vi "Corrected Flow Setpoint SI.vi"(7 "Set? (F:Read)":bool, 8 "Error In":errorcluster, 9 "Flow Setpoint (0 l/min)":dbl[unit], 10 "Channel (0)":i32, 11 "VISA resource name":refnum<visa-resource-name>) -> (0 "Error Out":errorcluster, 1 "Flow Setpoint out":dbl[unit], 3 "dup VISA resource name":refnum<visa-resource-name>)   [LabVIEW 2011, in "MGC647C.lvlib"]
doc: "Read/Set corrected flow setpoint of a channel in SI unit."
uses:
  <instrlib>/MGC647C/MGC647C.lvlib
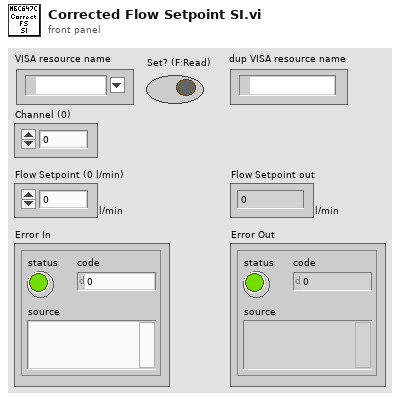
[diagram p1: front panel]
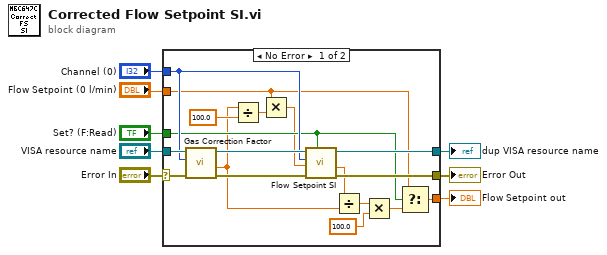
[diagram p0: block diagram]
diagram:
  n1 = case shown="No Error" "Error In" {
    selector: "Error In" -> [w25 w28]
    tunnel: "VISA resource name" -> [w26 w27]
    tunnel: [w21 w27] -> w7
    tunnel: [w20 w28] -> w6
    tunnel: "Set? (F:Read)" -> [w19 _]
    tunnel: "Flow Setpoint (0 l/min)" -> [w15 w29]
    tunnel: [w18 w29] -> w2
    tunnel: "Channel (0)" -> [w22 _]
    frame No Error {
      n2 = call <instrlib>:"Gas Correction Factor.vi"("Error In"=w25, "Channel (0)"=w22, "VISA resource name"=w26) -> ("Error Out"=w23:errorcluster, "Gas Correction Factor out"=w10:dbl, "dup VISA resource name"=w24:refnum<visa-resource-name>)  [unwired: 6 in]
      n3 = Divide(x=w10, y=100.0) -> (x/y=w16:dbl)
      n4 = Multiply(x=w15, y=w16) -> (x*y=w14:dbl[unit])
      n5 = call <instrlib>:"Flow Setpoint SI.vi"("Set? (F:Read)"=w19, "Error In"=w23, "Flow Setpoint (0 l/min)"=w14, "Channel (0)"=w22, "VISA resource name"=w24) -> ("Error Out"=w20:errorcluster, "Flow Setpoint out"=w11:dbl[unit], "dup VISA resource name"=w21:refnum<visa-resource-name>)  [unwired: 4 in]
      n6 = Divide(x=w11, y=w10) -> (x/y=w13:dbl[unit])
      n7 = Multiply(x=w13, y=100.0) -> (x*y=w9:dbl[unit])
      n8 = Select(t=w15, s=w19, f=w9) -> (s? t:f=w18:dbl[unit])
    }
    frame Error {
    }
  }
  "dup VISA resource name" <- w7
  "Error Out" <- w6
  "Flow Setpoint out" <- w2
